vi "SubPanel Guest-Core_Process.vi"(0 "FTW Actor Instance Configuration":string="{\n  \"Identity\": \"ActorName\",\n  \"InboxAddress\": \"inproc://*\",\n  \"PublisherAddress\": \"\",\n  \"LoggerAddress\": \"\",\n  \"DebugEnableInboxLogging\": false,\n  \"DebugEnableJobLogging\": false,\n  \"LauncherAddress\": \"\",\n  \"My Data\": false\n}", 11 "ErrorIn":errorcluster) -> (15 "Error":errorcluster)   [LabVIEW 2013, in "SubPanel Guest-Core.lvclass"]
uses:
  SubPanel Guest-Core.lvclass
  Actor/src/Message/Base/FTW-Message.lvclass
  SubPanel Guest-Core.lvclass/SubPanel Guest-Core.ctl
  Actor/src/Instance/FTW-ActorInstance.lvclass/FTW-ActorInstance.ctl
  Actor/src/JobSequencer/FTW-SEQ-Current.vi
  Actor/src/Instance/FTW-ActorInstance.lvclass
  Actor/src/Message/Request/FTW-Message-IncomingRequest.lvclass
panel:
  out "Heartbeat":bool
  out "Time":string
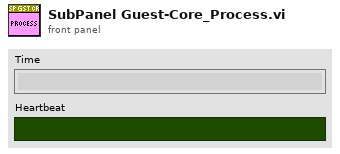
[diagram p1: front panel]
types:
  T1 = cluster{"Incoming Requests":refnum<event-registration>, "Local Messages":refnum<event-registration>, "Additional Registration Types":refnum<event-registration>}
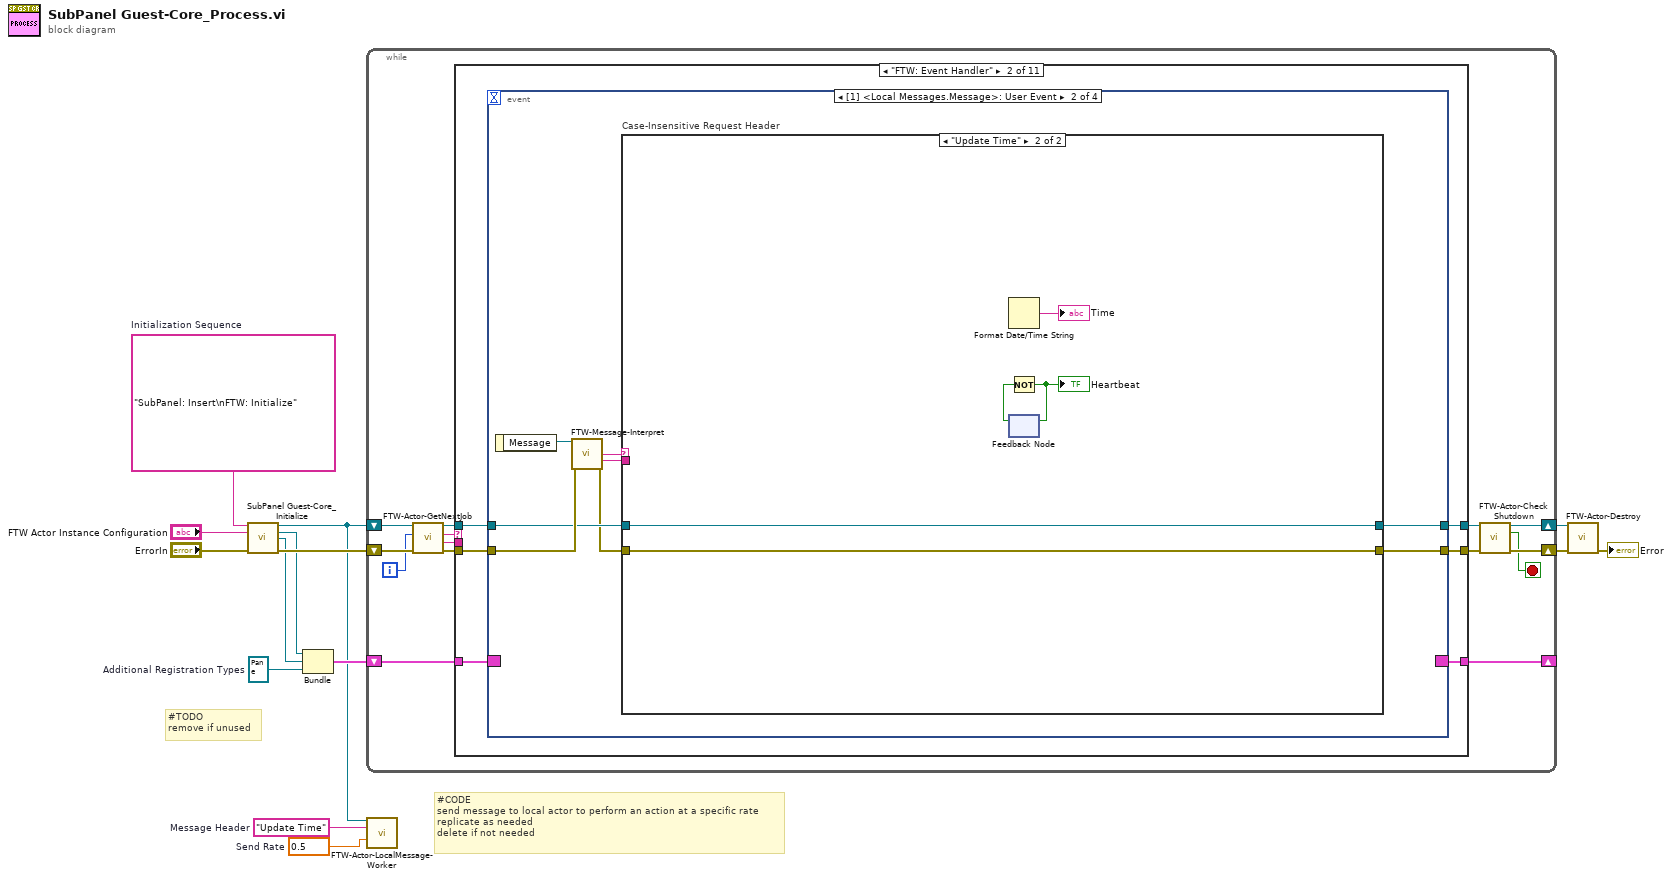
[diagram p0: block diagram]
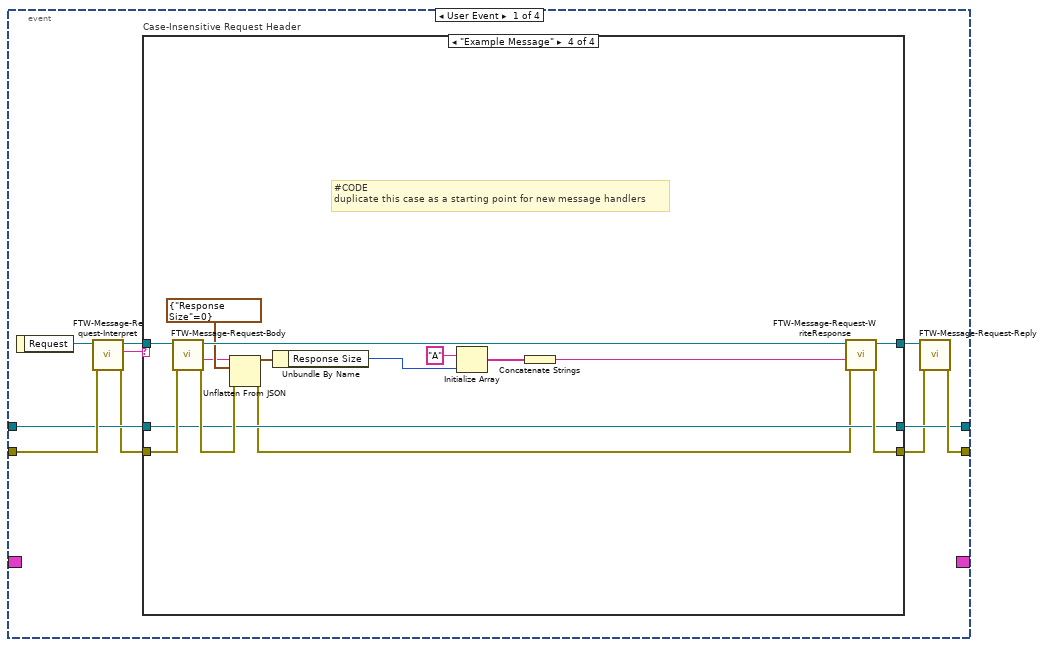
[diagram p3: hidden frame]
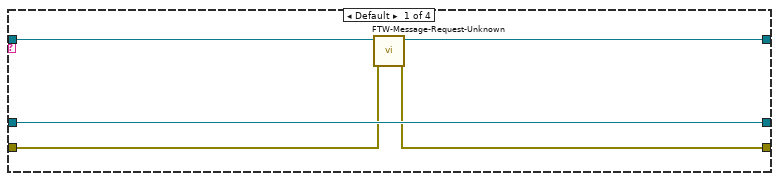
[diagram p4: hidden frame]
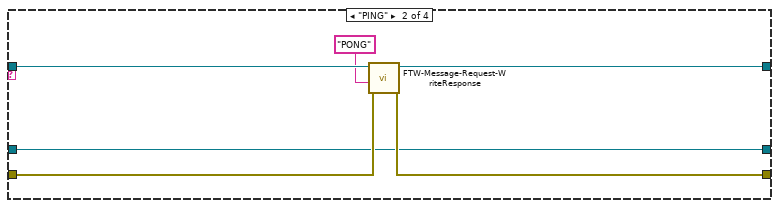
[diagram p5: hidden frame]
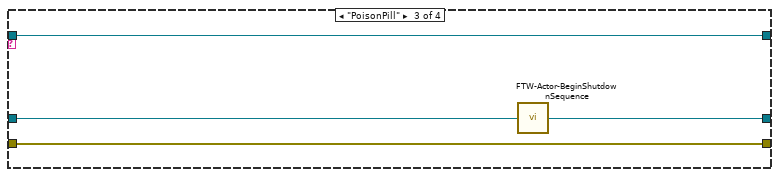
[diagram p6: hidden frame]
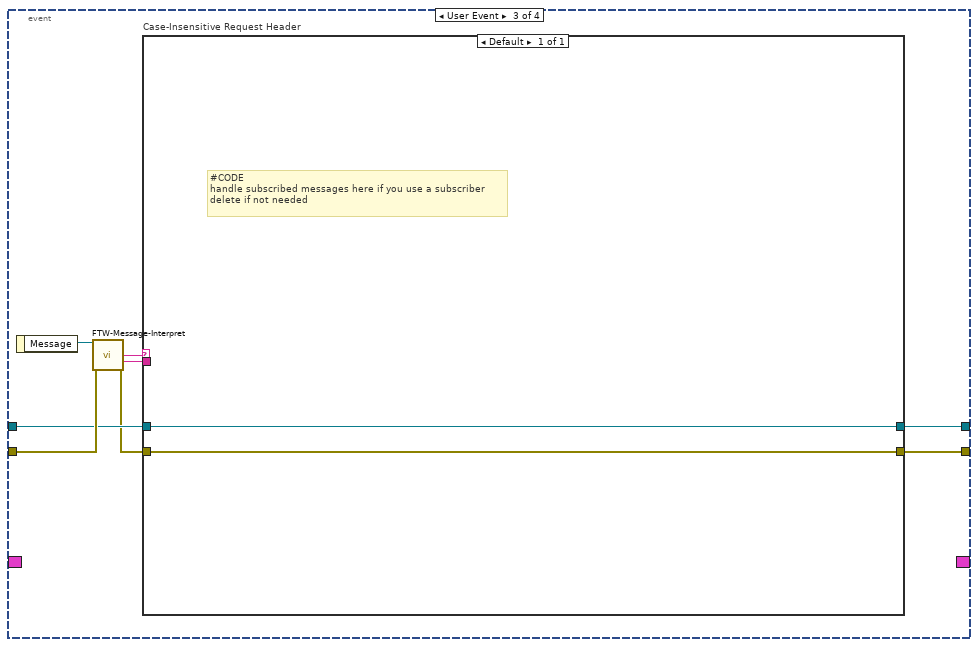
[diagram p8: hidden frame]
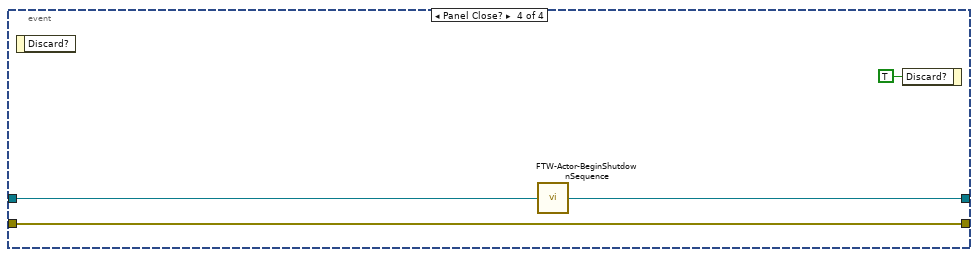
[diagram p9: hidden frame]
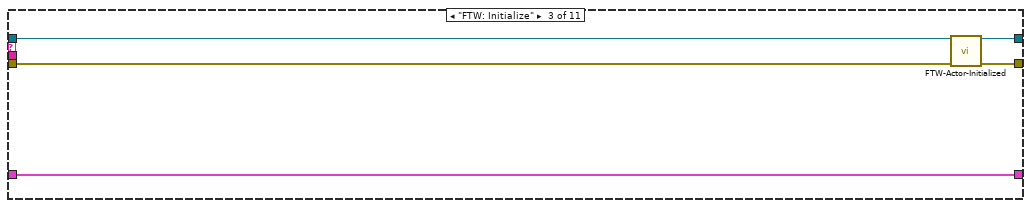
[diagram p10: hidden frame]
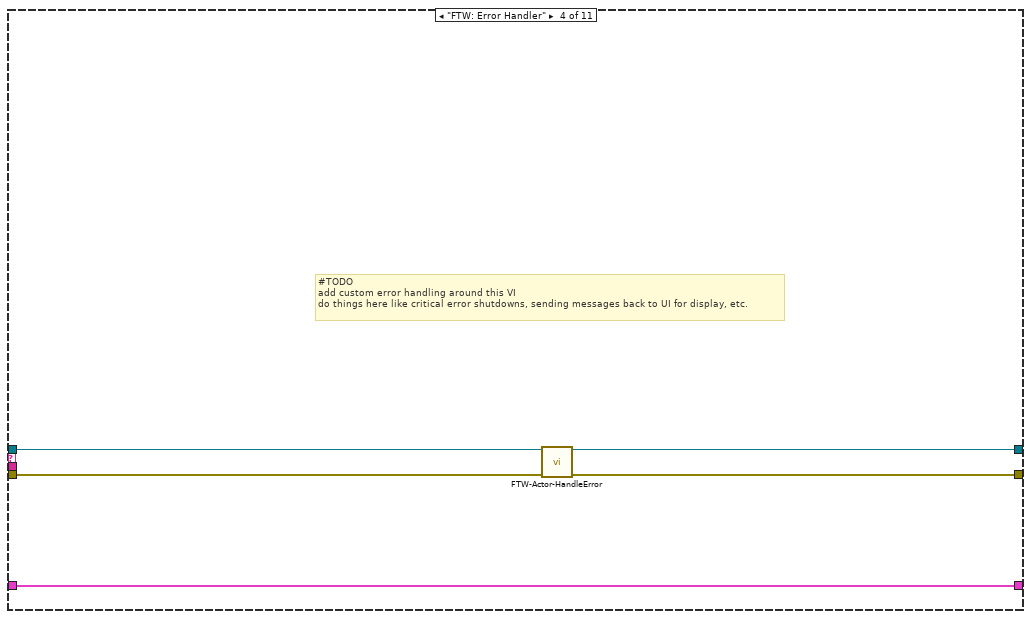
[diagram p11: hidden frame]
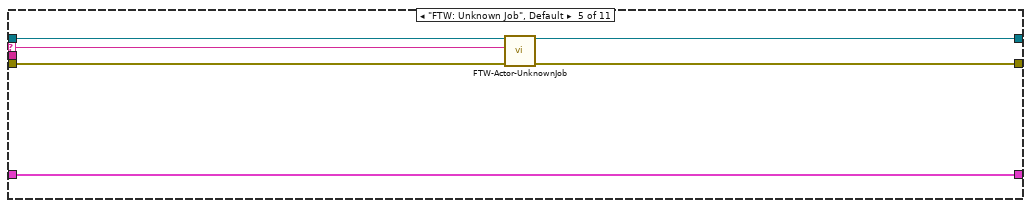
[diagram p12: hidden frame]
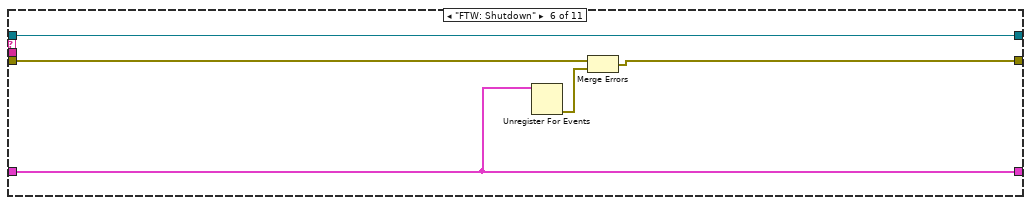
[diagram p13: hidden frame]
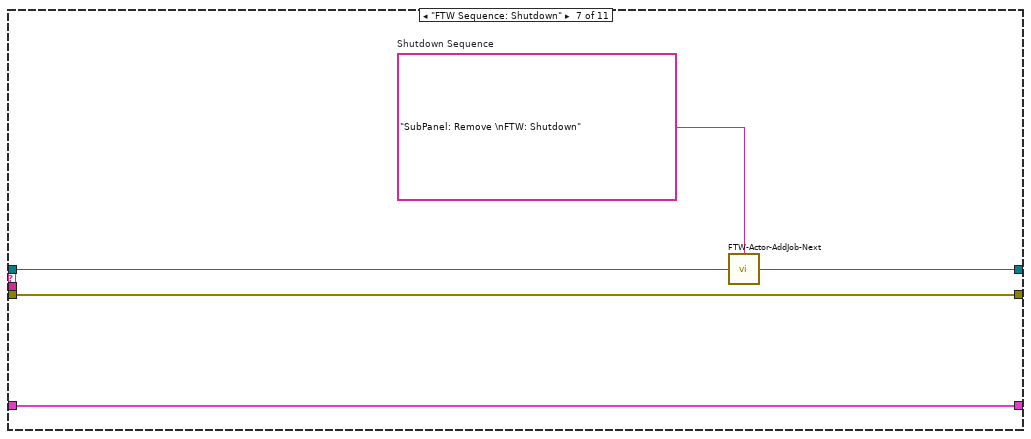
[diagram p14: hidden frame]
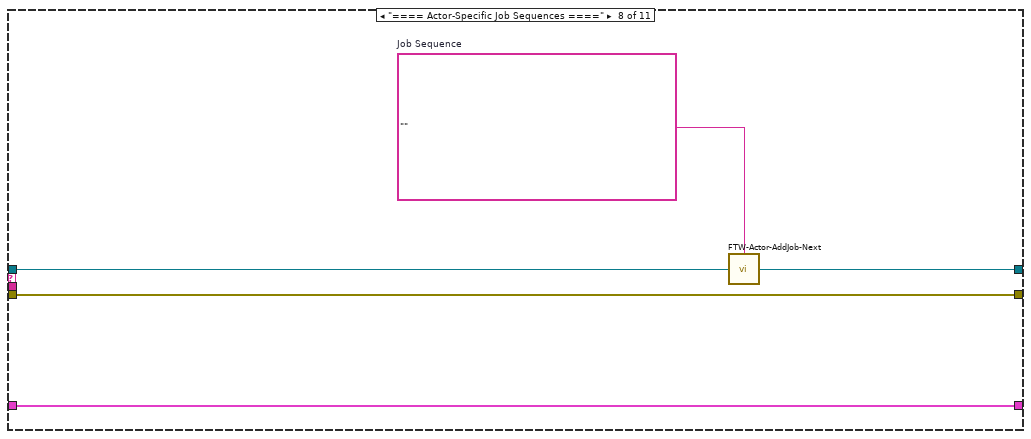
[diagram p15: hidden frame]
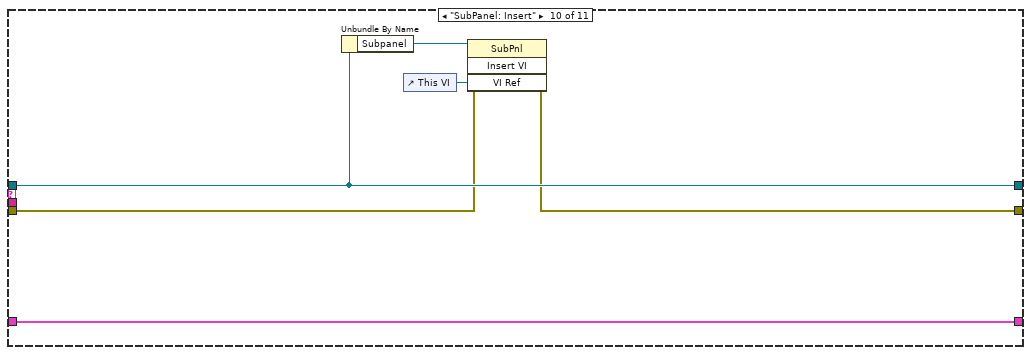
[diagram p17: hidden frame]
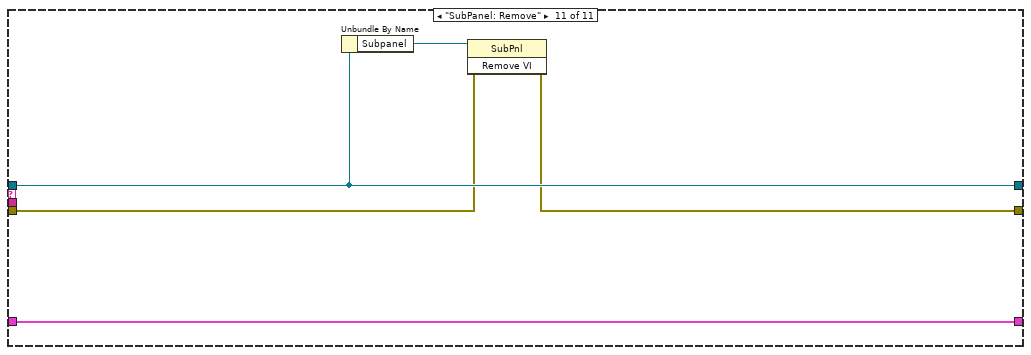
[diagram p18: hidden frame]
diagram:
  w2 = 0.5  # Send Rate
  w3 = "Update Time"  # Message Header
  w4 = refnum<event-registration> refnum  # Additional Registration Types
  w10 = "SubPanel: Insert\nFTW: Initialize"  # Initialization Sequence
  # "#CODE\nsend message to local actor to perform an action at a specific rate\nreplicate as needed\ndelete if not needed"
  # "#TODO\nremove if unused"
  n1 = call "SubPanel Guest-Core_Initialize.vi"("Initialization Sequence"=w10, "FTW Actor Instance Configuration"="FTW Actor Instance Configuration", "error in (no error)"="ErrorIn") -> ("Actor Template-Core out"=w1:refnum<class "SubPanel Guest-Core.lvclass">, "Incoming Requests"=w6:refnum<event-registration>, "Local Messages"=w5:refnum<event-registration>, "error out"=w11:errorcluster)  [unwired: 9 in]
  n2 = Bundle("Incoming Requests"=w6, "Local Messages"=w5, "Additional Registration Types"=w4) -> (w8:T1)  [unwired: 1 in]
  n3 = while {
    shift-right: [w18] -> w13
    shift-left: w11 -> [w25]
    shift-right: [w15] -> _
    shift-left: w8 -> [w28]
    shift-right: [w20] -> w14
    shift-left: w1 -> [w27]
    i -> [w16]
    stop <- w17 stop-if-true
    n4 = call "FTW-Actor-GetNextJob.vi"("error in"=w25, "Jobs Performed"=w16, "FTW Actor Instance"=w27) -> ("error out"=w24:errorcluster, "Job Data"=w22:string, "Job Name"=w23:string, "FTW Actor Instance out"=w26:refnum<class "SubPanel Guest-Core.lvclass">)  [unwired: 5 in]
    n5 = case shown="\"FTW: Event Handler\"" w23 {
      selector: w23 -> [_ _ _ _ w117 _ _ _ _ _ _]
      tunnel: [w30 w37 w107 w112 w120 w126 w131 w136 w140 w141 w147] -> w19
      tunnel: w24 -> [w30 w36 w110 w114 w121 w127 w131 w136 w140 w142 w148]
      tunnel: w28 -> [w31 w32 w111 w116 w122 w123 w132 w137 w139 w146 w151]
      tunnel: [w31 w35 w111 w116 w122 w123 w132 w137 w139 w146 w151] -> w15
      tunnel: w22 -> [_ _ _ _ _ _ _ _ _ _ _]
      tunnel: [w29 w34 w108 w113 w118 w124 w129 w134 w138 w145 w150] -> w21
      tunnel: w26 -> [w29 w33 w109 w115 w119 w124 w130 w135 w138 w145 w150]
      frame "==== Featherweight Framework Jobs ====" {
      }
      frame "FTW: Event Handler" {
        n6 = event shown="[1] <Local Messages.Message>: User Event" {
          selector: w32 -> [_ _ _ _]
          dyn-events: [_ _ _ _] -> w35
          timeout: _ -> [_ _ _ _]
          tunnel: [w46 w80 w95 w105] -> w37
          tunnel: w36 -> [w45 w84 w99 w105]
          tunnel: [w40 w81 w96 w103] -> w34
          tunnel: w33 -> [w44 w83 w98 w104]
          event User Event {
            n7 = event-data() -> ("Request"=w47:refnum<class "FTW-Message-IncomingRequest.lvclass">)  [unwired: 1 in]
            n8 = call "FTW-Message-Request-Interpret.vi"("error in"=w45, "FTW Incoming Request"=w47) -> ("error out"=w43:errorcluster, "Request Header"=w41:string, "FTW Incoming Request out"=w42:refnum<class "FTW-Message-IncomingRequest.lvclass">)  [unwired: 7 in]
            n9 = case "Case-Insensitive Request Header" shown="\"Example Message\"" w41 {
              tunnel: [w50 w56 w61 w74] -> w39
              tunnel: w43 -> [w51 w57 w61 w77]
              tunnel: [w52 w55 w62 w71] -> w40
              tunnel: w44 -> [w52 w55 w60 w71]
              tunnel: w42 -> [w49 w58 w59 w75]
              tunnel: [w48 w54 w59 w72] -> w38
              frame Default {
                n10 = call "FTW-Message-Request-Unknown.vi"("error in"=w51, "FTW Incoming Request"=w49) -> ("error out"=w50:errorcluster, "FTW Incoming Request Out"=w48:refnum<class "FTW-Message-IncomingRequest.lvclass">)  [unwired: 8 in]
              }
              frame "PING" {
                n11 = call "FTW-Message-Request-WriteResponse.vi"("error in"=w57, "Response Body"="PONG" ("Response Header"), "FTW Incoming Request"=w58) -> ("error out"=w56:errorcluster, "FTW Incoming Request out"=w54:refnum<class "FTW-Message-IncomingRequest.lvclass">)  [unwired: 7 in]
              }
              frame "PoisonPill" {
                n12 = call "FTW-Actor-BeginShutdownSequence.vi"("FTW Actor Instance"=w60) -> ("FTW Actor Instance out"=w62:refnum<class "SubPanel Guest-Core.lvclass">)  [unwired: 3 in]
              }
              frame "Example Message" {
                # "#CODE\nduplicate this case as a starting point for new message handlers"
                n13 = call "FTW-Message-Request-Body.vi"("error in"=w77, "FTW Incoming Request"=w75) -> ("error out"=w76:errorcluster, "Request Body"=w68:string, "FTW Incoming Request out"=w73:refnum<class "FTW-Message-IncomingRequest.lvclass">)  [unwired: 7 in]
                n14 = Unflatten From JSON(JSON string=w68, type and defaults=cluster{"Response Size":i32} {"Response Size"=0}, error in (no error)=w76) -> (value=w67:cluster{"Response Size":i32}, error out=w70:errorcluster)  [unwired: 4 in]
                n15 = Unbundle By Name(w67) -> ("Response Size"=w66:i32)
                n16 = Initialize Array("A", w66) -> (w64:string[])
                n17 = Concatenate Strings(w64) -> (w63:string)
                n18 = call "FTW-Message-Request-WriteResponse.vi"("error in"=w70, "Response Body"=w63, "FTW Incoming Request"=w73) -> ("error out"=w74:errorcluster, "FTW Incoming Request out"=w72:refnum<class "FTW-Message-IncomingRequest.lvclass">)  [unwired: 7 in]
              }
            }
            n19 = call "FTW-Message-Request-Reply.vi"("error in"=w39, "FTW Incoming Request"=w38) -> ("error out"=w46:errorcluster)  [unwired: 8 in, 1 out]
          }
          event User Event {
            n20 = event-data() -> ("Message"=w85:refnum<class "FTW-Message.lvclass">)  [unwired: 1 in]
            n21 = call-dynamic "FTW-Message-Interpret.vi"("FTW Message"=w85, "error in"=w84) -> ("Message Header"=w79:string, "Message Body"=w78:string, "error out"=w82:errorcluster)  [unwired: 9 in, 2 out]
            n22 = case "Case-Insensitive Request Header" shown="\"Update Time\"" w79 {
              tunnel: [w86 w91] -> w80
              tunnel: w82 -> [w86 w91]
              tunnel: [w87 w92] -> w81
              tunnel: w83 -> [w87 w92]
              tunnel: w78 -> [_ _]
              frame Default {
                # "#CODE\nhandle local messages here\ndelete if not needed"
              }
              frame "Update Time" {
                n23 = Format Date/Time String() -> (date/time string=→"Time":string)  [unwired: 3 in]
                n24 = feedback #1() -> (w88:bool)  [unwired: 1 in]
                n25 = Not(x=w88) -> (.not. x?=w89:bool)
                "Heartbeat" <- w89
                n26 = feedback-in #1(w89) -> ()
              }
            }
          }
          event User Event {
            n27 = event-data() -> ("Message"=w100:refnum<class "FTW-Message.lvclass">)  [unwired: 1 in]
            n28 = call-dynamic "FTW-Message-Interpret.vi"("FTW Message"=w100, "error in"=w99) -> ("Message Header"=w94:string, "Message Body"=w93:string, "error out"=w97:errorcluster)  [unwired: 9 in, 2 out]
            n29 = case "Case-Insensitive Request Header" shown="Default" w94 {
              tunnel: [w101] -> w95
              tunnel: w97 -> [w101]
              tunnel: [w102] -> w96
              tunnel: w98 -> [w102]
              tunnel: w93 -> [_]
              frame Default {
                # "#CODE\nhandle subscribed messages here if you use a subscriber\ndelete if not needed"
              }
            }
          }
          event Panel Close? {
            n30 = event-data() -> ()  [unwired: 1 in, 1 out]
            n31 = call "FTW-Actor-BeginShutdownSequence.vi"("FTW Actor Instance"=w104) -> ("FTW Actor Instance out"=w103:refnum<class "SubPanel Guest-Core.lvclass">)  [unwired: 3 in]
            n32 = event-data("Discard?"=TRUE) -> ()  [unwired: 1 in, 1 out]
          }
        }
      }
      frame "FTW: Initialize" {
        n33 = call-dynamic "FTW-Actor-Initialized.vi"("FTW Actor Instance"=w109, "error in"=w110) -> ("FTW Actor Instance out"=w108:refnum<class "SubPanel Guest-Core.lvclass">, "error out"=w107:errorcluster)  [unwired: 12 in]
      }
      frame "FTW: Error Handler" {
        # "#TODO\nadd custom error handling around this VI\ndo things here like critical error shutdowns, sending messages back to UI for display, etc."
        n34 = call-dynamic "FTW-Actor-HandleError.vi"("FTW Actor Instance"=w115, "error in"=w114) -> ("FTW Actor Instance out"=w113:refnum<class "SubPanel Guest-Core.lvclass">, "error out"=w112:errorcluster)  [unwired: 11 in, 1 out]
      }
      frame "FTW: Unknown Job", Default {
        n35 = call-dynamic "FTW-Actor-UnknownJob.vi"("FTW Actor Instance"=w119, "Unknown Job"=w117, "error in"=w121) -> ("FTW Actor Instance out"=w118:refnum<class "SubPanel Guest-Core.lvclass">, "error out"=w120:errorcluster)  [unwired: 11 in]
      }
      frame "FTW: Shutdown" {
        n36 = Unregister For Events(event registration refnum=w123) -> (error out=w125:errorcluster)  [unwired: 1 in]
        n37 = Merge Errors(w127, w125) -> (w126:errorcluster)
      }
      frame "FTW Sequence: Shutdown" {
        w128 = "SubPanel: Remove \nFTW: Shutdown"  # Shutdown Sequence
        n38 = call "FTW-Actor-AddJob-Next.vi"("Add Next in Job Queue"=w128, "FTW Actor Instance"=w130) -> ("FTW Actor Instance out"=w129:refnum<class "SubPanel Guest-Core.lvclass">)  [unwired: 2 in]
      }
      frame "==== Actor-Specific Job Sequences ====" {
        w133 = ""  # Job Sequence
        n39 = call "FTW-Actor-AddJob-Next.vi"("Add Next in Job Queue"=w133, "FTW Actor Instance"=w135) -> ("FTW Actor Instance out"=w134:refnum<class "SubPanel Guest-Core.lvclass">)  [unwired: 2 in]
      }
      frame "==== Actor-Specific Jobs ====" {
      }
      frame "SubPanel: Insert" {
        n40 = Unbundle By Name(w145) -> ("Subpanel"=w144:refnum<vi>)
        n41 = control-ref of="This VI"() -> (w143:refnum<vi>)
        n42 = invoke class="SubPnl" method="Insert VI"(reference=w144, error in=w142, "VI Ref"=w143) -> (error out=w141:errorcluster)  [unwired: 1 in, 3 out]
      }
      frame "SubPanel: Remove" {
        n43 = Unbundle By Name(w150) -> ("Subpanel"=w149:refnum<vi>)
        n44 = invoke class="SubPnl" method="Remove VI"(reference=w149, error in=w148) -> (error out=w147:errorcluster)  [unwired: 1 in, 2 out]
      }
    }
    n45 = call "FTW-Actor-CheckShutdown.vi"("FTW Actor Instance"=w21, "error in"=w19) -> ("FTW Actor Instance out"=w20:refnum<class "SubPanel Guest-Core.lvclass">, "Shutdown?"=w17:bool, "error out"=w18:errorcluster)  [unwired: 11 in]
  }
  n46 = call-dynamic "FTW-Actor-LocalMessage-Worker.vi"("FTW-ActorInstance In"=w1, "Message Header"=w3, "Send Rate"=w2) -> ()  [unwired: 12 in, 1 out]
  n47 = call-dynamic "FTW-Actor-Destroy.vi"("FTW Actor Instance"=w14, "error in"=w13) -> ("error out"=→"Error":errorcluster)  [unwired: 13 in]
